vi "CoboltLaser_OutputPowerRead.vi"(0 "ComPort":refnum<visa-resource-name>, 7 "CheckResponse":bool=TRUE, 11 "ErrorIn":errorcluster) -> (4 "ComPortOut":refnum<visa-resource-name>, 6 "OutputPower":dbl format="%.4g", 15 "ErrorOut":errorcluster)   [LabVIEW 2019]
doc: "Use this template to build a VI to use as a subVI."
panel:
  out "ResponseOK":bool
  out "Response":string
  # "(W)"
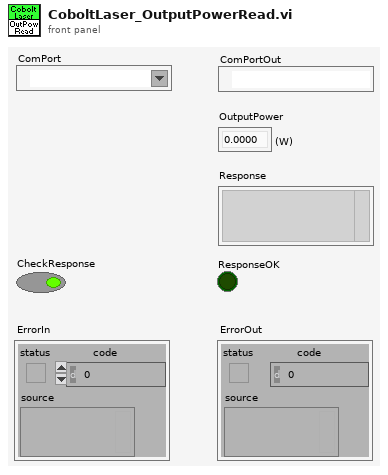
[diagram p1: front panel]
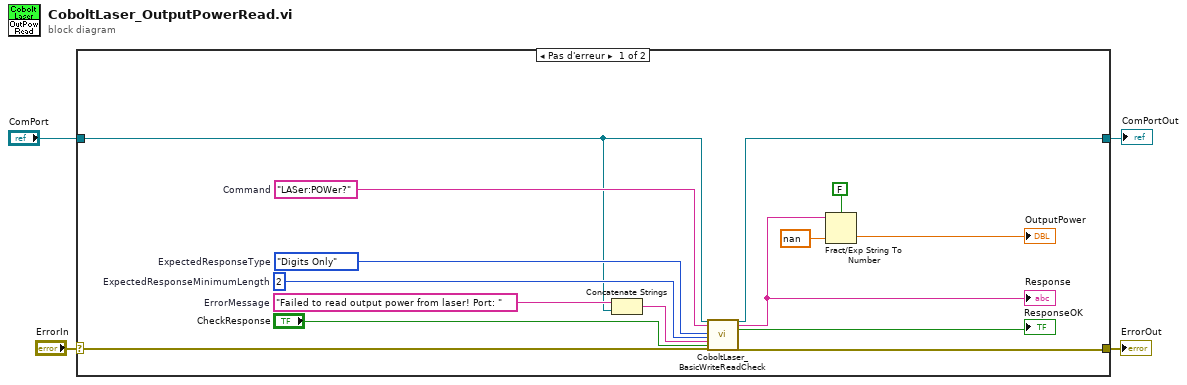
[diagram p0: block diagram]
diagram:
  n1 = case shown="Pas d'erreur" "ErrorIn" {
    selector: "ErrorIn" -> [w19 w21]
    tunnel: [w18 w21] -> w3
    tunnel: "ComPort" -> [w8 w20]
    tunnel: [w7 w20] -> w1
    frame No Error {
      w15 = 2  # ExpectedResponseMinimumLength
      w16 = enum16{"Any", "Digits Only", "Non-Digits Only"}."Digits Only"  # ExpectedResponseType
      w12 = "Failed to read output power from laser! Port: "  # ErrorMessage
      w17 = "LASer:POWer?"  # Command
      n2 = Concatenate Strings(w12, w8) -> (w11:string)
      n3 = call <userlib>:"CoboltLaser_BasicWriteReadCheck.vi"("ComPort"=w8, "Command"=w17, "ExpectedResponseType"=w16, "ExpectedResponseMinimumLength"=w15, "ErrorMessage"=w11, "GenerateError"="CheckResponse", "error in (no error)"=w19) -> ("ComPortOut"=w7:refnum<visa-resource-name>, "Response"=w10:string, "ResponseOK"=→"ResponseOK":bool, "error out"=w18:errorcluster)  [unwired: 17 in]
      "Response" <- w10
      n4 = Fract/Exp String To Number(use system decimal point (T)=FALSE, string=w10, default (0 dbl)=nan ("default (0 DBL)")) -> (number=→"OutputPower":dbl)  [unwired: 1 in, 1 out]
    }
    frame Error {
    }
  }
  "ErrorOut" <- w3
  "ComPortOut" <- w1
